vi "Create RPC Client Method.vi"(8 "error in (no error)":errorcluster, 10 "RPC Method Parameters":T1, 11 "Library":refnum<vi>) -> (0 "error out":errorcluster, 2 "Newly created ?":bool, 3 "Library":refnum<vi>)   [LabVIEW 2019, in "gRPC Template Creation Utility.lvlib"]
uses:
  gRPC Template Creation Utility.lvlib
  TypeDefs/RPC Method Parameters.ctl
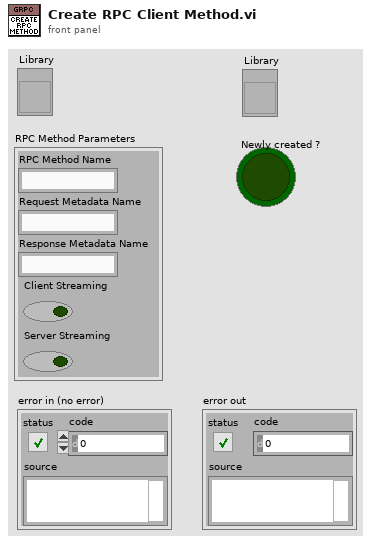
[diagram p1: front panel]
types:
  T1 = typedef "gRPC Template Creation Utility.lvlib/RPC Method Parameters.ctl" = cluster{"RPC Method Name":string, "Request Metadata Name":string, "Response Metadata Name":string, "Client Streaming":bool, "Server Streaming":bool}
  T2 = enum32{"invalid VI type", "Standard VI", "Control VI", "Global VI", "Polymorphic VI", "Configuration VI", "SubSystem", "Facade VI", "Method VI"}
  T3 = typedef "gRPC Template Creation Utility.lvlib/RPC Method Types.ctl" = enum16{"Unary", "Server Stream", "Client Stream", "Bidirectional Stream"}
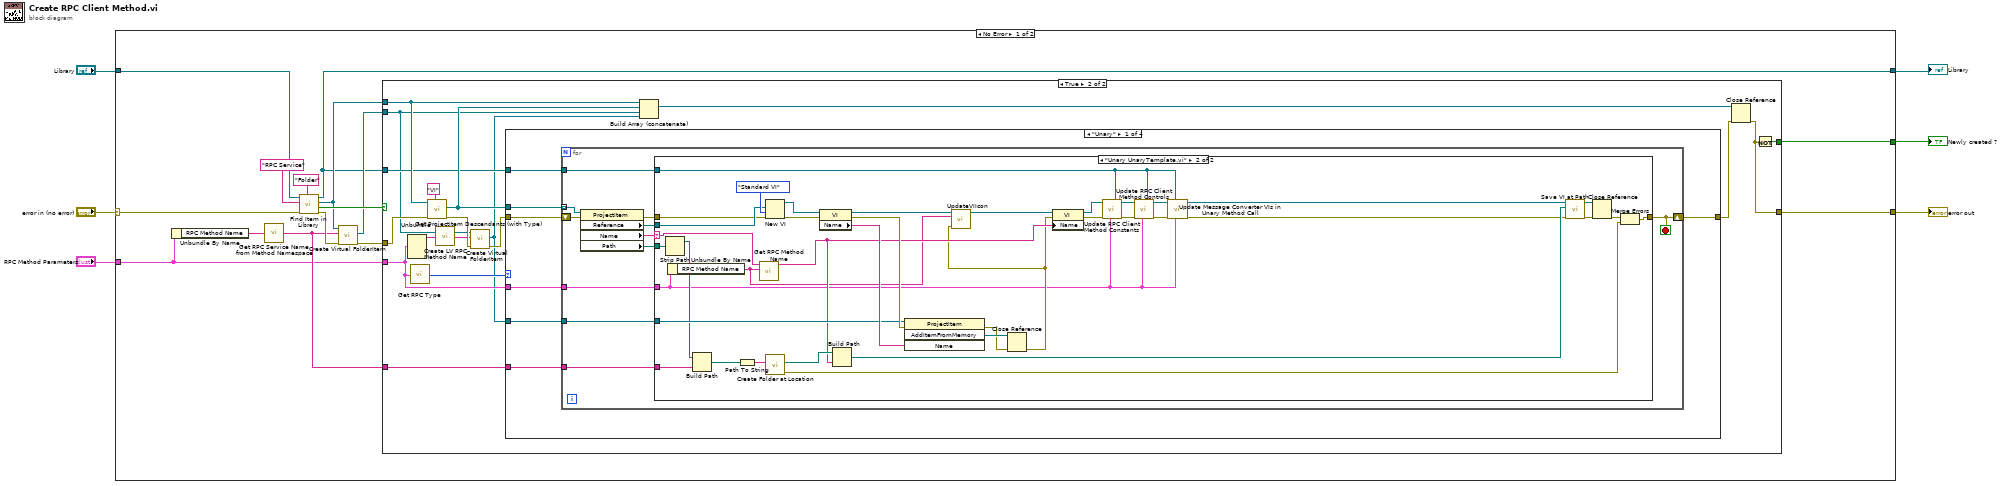
[diagram p0: block diagram]
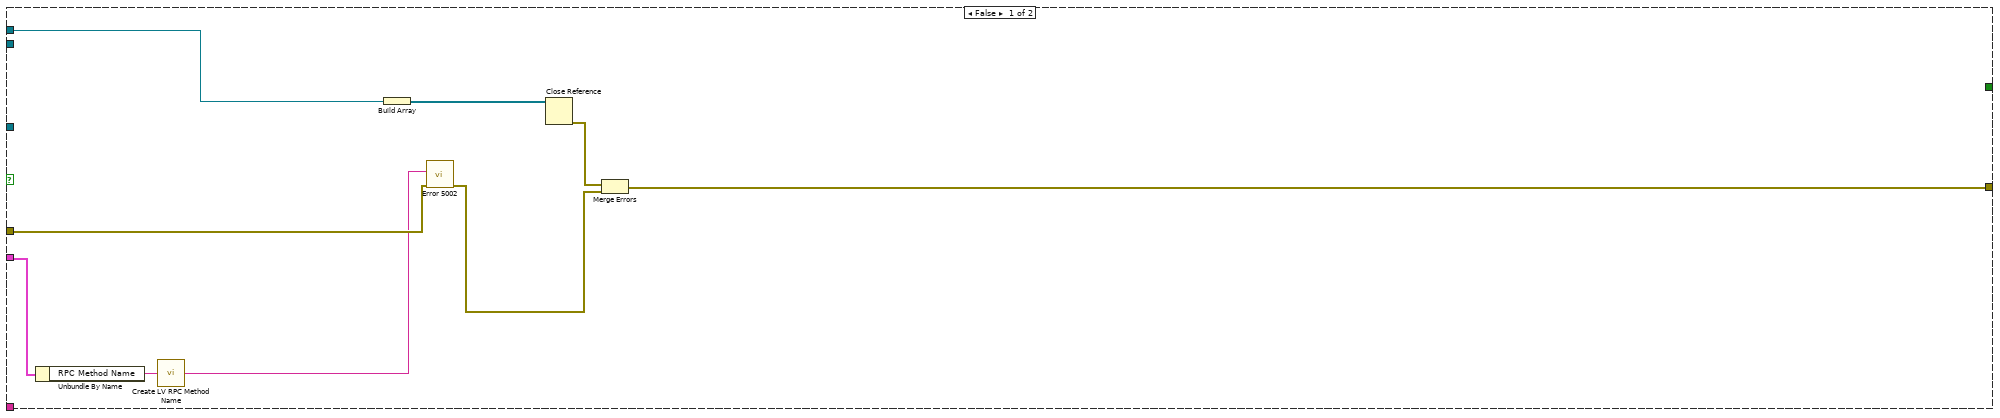
[diagram p2: hidden frame]
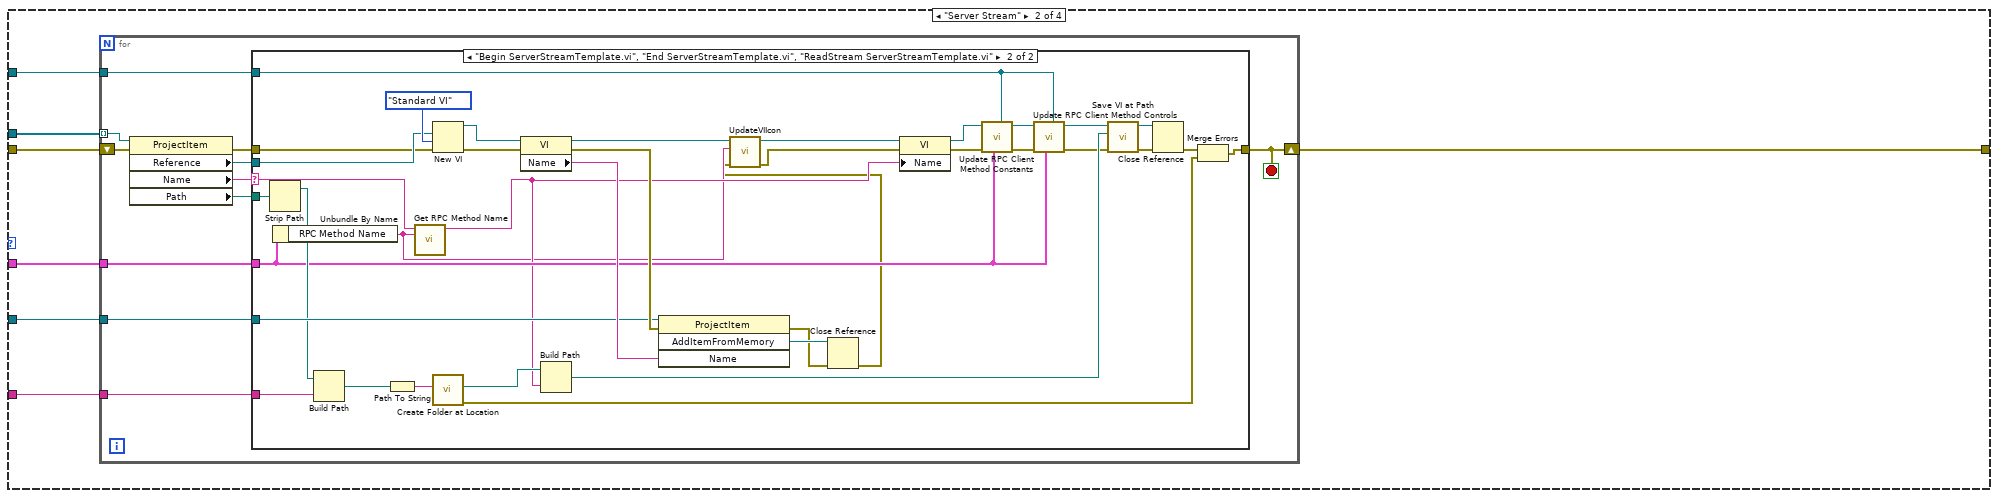
[diagram p4: hidden frame]
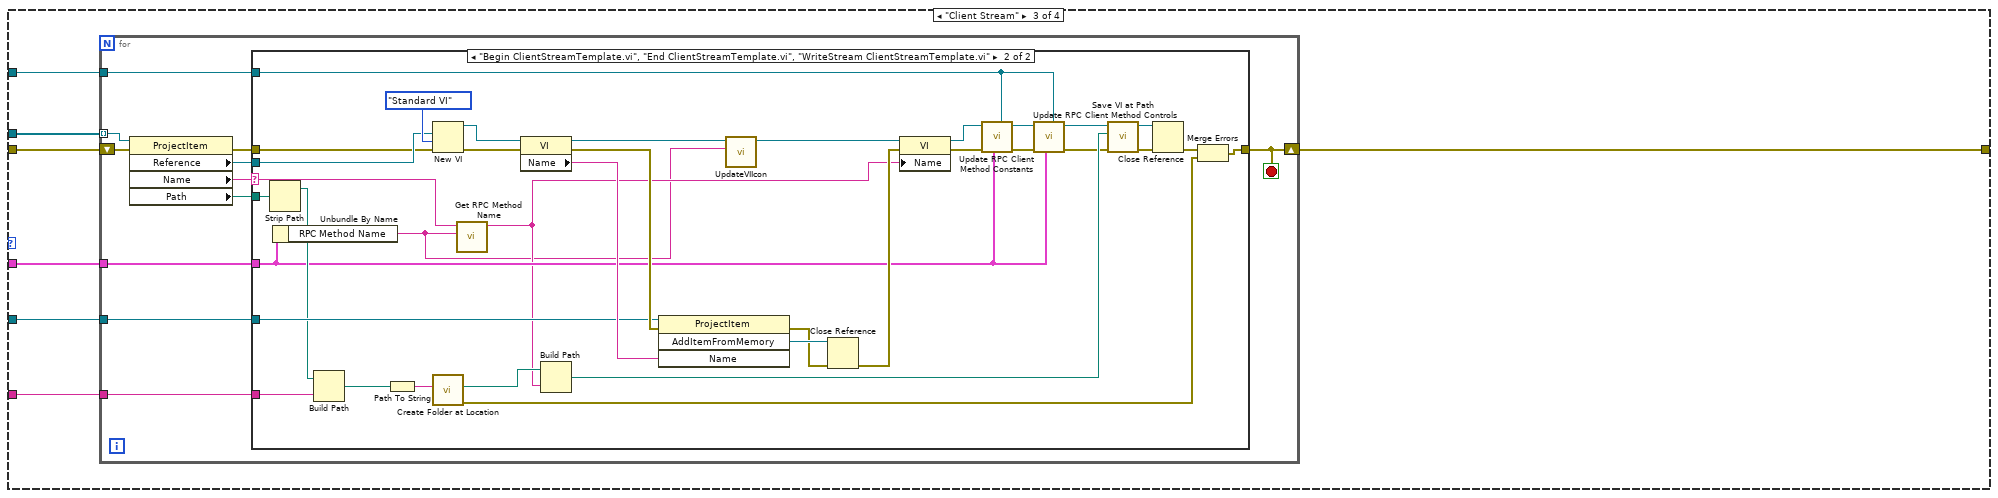
[diagram p6: hidden frame]
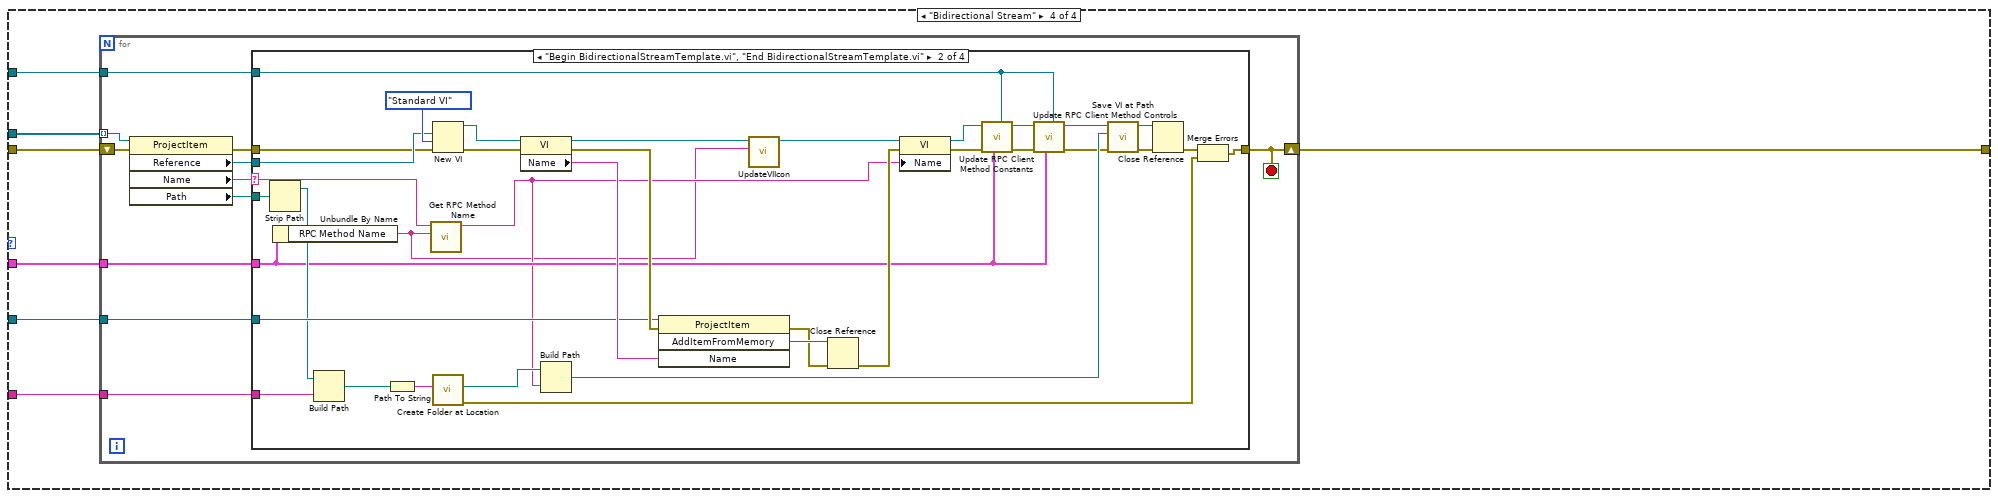
[diagram p8: hidden frame]
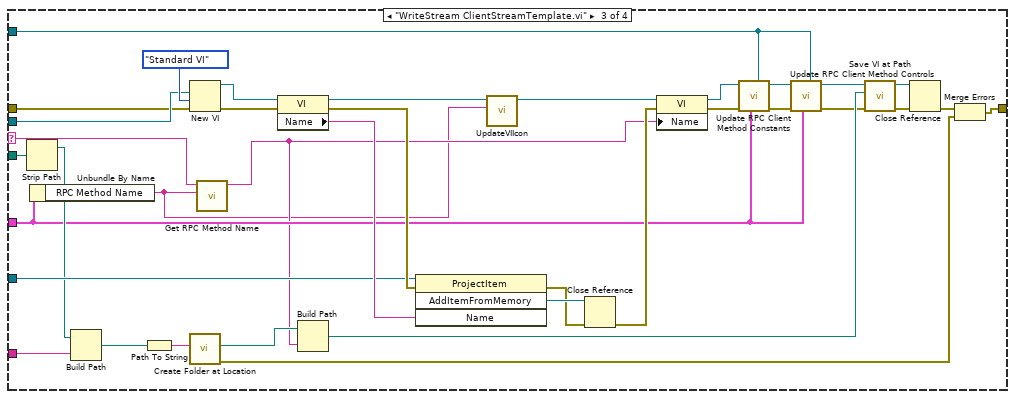
[diagram p10: hidden frame]
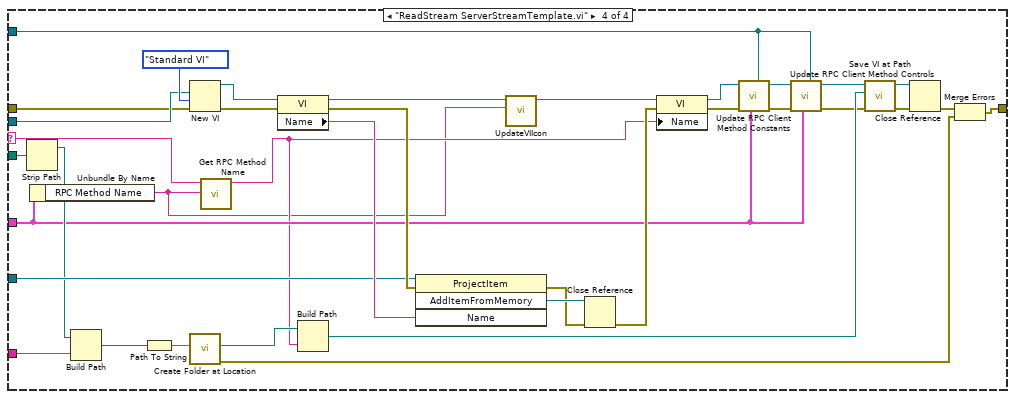
[diagram p11: hidden frame]
diagram:
  n1 = case shown="No Error" "error in (no error)" {
    selector: "error in (no error)" -> [w18 w345]
    tunnel: "Library" -> [w8 w344]
    tunnel: [w19 w345] -> w5
    tunnel: [w7 w344] -> w3
    tunnel: [w17 _] -> w2
    tunnel: "RPC Method Parameters" -> [w9 _]
    frame No Error {
      n2 = Unbundle By Name(w9) -> ("RPC Method Name"=w15:string)
      n3 = call "Get RPC Service Name from Method Namespace.vi"("RPC Method Name"=w15) -> ("RPC Service Name"=w10:string)
      n4 = call "Find Item in Library.vi"("Item Type"="Folder", "error in (no error)"=w18, "Item Name"="RPC Service", "Library item in"=w8) -> ("error out"=w14:errorcluster, "Found?"=w16:bool, "Project Item (Library Item)"=w12:refnum<vi>, "Library item out"=w7:refnum<vi>)  [unwired: 4 in]
      n5 = call "Create Virtual FolderItem.vi"("error in (no error)"=w14, "Folder Name"=w10, "ProjectItem in"=w12) -> ("error out"=w13:errorcluster, "FolderItem reference out"=w11:refnum<vi>)  [unwired: 5 in, 2 out]
      n6 = case shown="True" w16 {
        tunnel: w12 -> [w29 w41]
        tunnel: w13 -> [w30 w42]
        tunnel: [w25 w48] -> w19
        tunnel: [_ w47] -> w17
        tunnel: w11 -> [_ w35]
        tunnel: w10 -> [_ w40]
        tunnel: w9 -> [w24 w34]
        tunnel: w7 -> [_ w38]
        frame False {
          n7 = Unbundle By Name(w24) -> ("RPC Method Name"=w23:string)
          n8 = call "Create LV RPC Method Name.vi"("Proto Parser RPC Method Name in"=w23) -> ("LV RPC Method Name out"=w22:string)
          n9 = Build Array(w29) -> (w28:refnum<vi>[])
          n10 = call "Error 5002.vi"("error in (no error)"=w30, "Method Name"=w22) -> ("error out"=w27:errorcluster)  [unwired: 9 in]
          n11 = Close Reference(reference=w28) -> (error out=w26:errorcluster)  [unwired: 1 in]
          n12 = Merge Errors(w26, w27) -> (w25:errorcluster)
        }
        frame True {
          n13 = Unbundle(w34) -> ("RPC Method Name"=w32:string)  [unwired: 4 out]
          n14 = call "Get RPC Type.vi"("RPC Method Parameters"=w34) -> ("RPC Type"=w39:T3)
          n15 = call "Get ProjectItem Descendants (with Type).vi"("Type"="VI", "error in (no error)"=w42, "ProjectItem in"=w41) -> ("error out"=w37:errorcluster, "All Descendents"=w44:refnum<vi>[])  [unwired: 6 in, 1 out]
          n16 = call "Create LV RPC Method Name.vi"("Proto Parser RPC Method Name in"=w32) -> ("LV RPC Method Name out"=w31:string)
          n17 = call "Create Virtual FolderItem.vi"("error in (no error)"=w37, "Folder Name"=w31, "ProjectItem in"=w35) -> ("error out"=w36:errorcluster, "FolderItem reference out"=w33:refnum<vi>)  [unwired: 5 in, 2 out]
          n18 = case shown="\"Unary\"" w39 {
            tunnel: w44 -> [w55 w112 w168 w223]
            tunnel: w36 -> [w54 w111 w167 w222]
            tunnel: [w53 w110 w166 w221] -> w43
            tunnel: w33 -> [w52 w109 w165 w220]
            tunnel: w40 -> [w51 w108 w164 w219]
            tunnel: w34 -> [w50 w107 w163 w218]
            tunnel: w38 -> [w49 w106 w162 w217]
            frame "Unary" {
              n19 = for {
                tunnel: w55 -> [w66] mode=indexing
                tunnel: w52 -> [w61]
                shift-right: [w59] -> w53
                shift-left: w54 -> [w65]
                tunnel: w51 -> [w58]
                tunnel: w50 -> [w57]
                tunnel: w49 -> [w56]
                stop <- w59 stop-if-true
                n20 = property class="ProjectItem"(reference=w66, error in=w65) -> (error out=w60:errorcluster, "Reference"=w63:refnum<vi>, "Name"=w64:string, "Path"=w62:path)  [unwired: 1 out]
                n21 = case shown="\"Unary UnaryTemplate.vi\"" w64 {
                  selector: w64 -> [_ w79]
                  tunnel: w63 -> [_ w95]
                  tunnel: w62 -> [_ w91]
                  tunnel: w61 -> [_ w94]
                  tunnel: w60 -> [w67 w93]
                  tunnel: [w67 w85] -> w59
                  tunnel: w58 -> [_ w89]
                  tunnel: w57 -> [_ w69]
                  tunnel: w56 -> [_ w68]
                  frame "None", Default {
                  }
                  frame "Unary UnaryTemplate.vi" {
                    n22 = Strip Path(path=w91) -> (stripped path=w90:path)  [unwired: 1 out]
                    n23 = Unbundle By Name(w69) -> ("RPC Method Name"=w75:string)
                    n24 = Build Path(base path=w90, name or relative path=w89) -> (appended path=w88:path)
                    n25 = Path To String(path=w88) -> (string=w87:string)
                    n26 = call "Get RPC Method Name.vi"("RPC Method Name"=w75, "Template VI Name"=w79) -> ("RPC VI Name"=w78:string)  [unwired: 8 in, 1 out]
                    n27 = New VI(8:w93, 9:T2."Standard VI" ("vi type (standard vi)"), 10:w95) -> (0:w102:errorcluster, 3:w104:refnum<vi>)  [unwired: 1 in, 3 out]
                    n28 = call "Create Folder at Location.vi"("Path"=w87) -> ("Error Out"=w84:errorcluster, "Full path out"=w86:path)  [unwired: 8 in, 1 out]
                    n29 = property class="VI"(reference=w104, error in=w102) -> (reference out=w77:refnum<vi>, error out=w101:errorcluster, "Name"=w105:string)
                    n30 = Build Path(base path=w86, name or relative path=w78) -> (appended path=w100:path)
                    n31 = invoke class="ProjectItem" method="AddItemFromMemory"(reference=w94, error in=w101, "Name"=w105) -> (error out=w96:errorcluster, "AddItemFromMemory"=w97:refnum<vi>)  [unwired: 1 in, 2 out]
                    n32 = Close Reference(reference=w97, error in (no error)=w96) -> (error out=w74:errorcluster)
                    n33 = call "UpdateVIIcon.vi"("error in (no error)"=w74, "Method Name"=w75, "VI in"=w77) -> ("VI out"=w76:refnum<vi>)  [unwired: 7 in, 1 out]
                    n34 = property class="VI"(reference=w76, error in=w74, "Name"=w78) -> (reference out=w81:refnum<vi>, error out=w83:errorcluster)
                    n35 = call "Update RPC Client Method Constants.vi"("Library"=w68, "RPC Method Parameters"=w69, "error in (no error)"=w83, "VI in"=w81) -> ("error out"=w82:errorcluster, "VI out"=w80:refnum<vi>)  [unwired: 6 in]
                    n36 = call "Update RPC Client Method Controls.vi"("Library"=w68, "RPC Method Parameters"=w69, "error in (no error)"=w82, "VI in"=w80) -> ("error out"=w71:errorcluster, "VI out"=w73:refnum<vi>)  [unwired: 6 in]
                    n37 = call "Update Message Converter VIs in Unary Method Call.vi"("RPC Method Parameters"=w69, "Library"=w68, "error in (no error)"=w71, "VI in"=w73) -> ("error out"=w70:errorcluster, "VI out"=w72:refnum<vi>)  [unwired: 6 in]
                    n38 = call "Save VI at Path.vi"("error in (no error)"=w70, "Path"=w100, "VI in"=w72) -> ("error out"=w99:errorcluster, "VI out"=w98:refnum<vi>)  [unwired: 6 in, 1 out]
                    n39 = Close Reference(reference=w98, error in (no error)=w99) -> (error out=w92:errorcluster)
                    n40 = Merge Errors(w92, w84) -> (w85:errorcluster)
                  }
                }
              }
            }
            frame "Server Stream" {
              n41 = for {
                tunnel: w112 -> [w123] mode=indexing
                tunnel: w109 -> [w118]
                shift-right: [w116] -> w110
                shift-left: w111 -> [w122]
                tunnel: w108 -> [w115]
                tunnel: w107 -> [w114]
                tunnel: w106 -> [w113]
                stop <- w116 stop-if-true
                n42 = property class="ProjectItem"(reference=w123, error in=w122) -> (error out=w117:errorcluster, "Reference"=w120:refnum<vi>, "Name"=w121:string, "Path"=w119:path)  [unwired: 1 out]
                n43 = case shown="\"Begin ServerStreamTemplate.vi\", \"End ServerStreamTemplate.vi\", \"ReadStream ServerStreamTemplate.vi\"" w121 {
                  selector: w121 -> [_ w130]
                  tunnel: w120 -> [_ w151]
                  tunnel: w119 -> [_ w147]
                  tunnel: w118 -> [_ w150]
                  tunnel: w117 -> [w124 w149]
                  tunnel: [w124 w141] -> w116
                  tunnel: w115 -> [_ w145]
                  tunnel: w114 -> [_ w133]
                  tunnel: w113 -> [_ w132]
                  frame "None", Default {
                  }
                  frame "Begin ServerStreamTemplate.vi", "End ServerStreamTemplate.vi", "ReadStream ServerStreamTemplate.vi" {
                    n44 = Strip Path(path=w147) -> (stripped path=w146:path)  [unwired: 1 out]
                    n45 = Unbundle By Name(w133) -> ("RPC Method Name"=w127:string)
                    n46 = Build Path(base path=w146, name or relative path=w145) -> (appended path=w144:path)
                    n47 = Path To String(path=w144) -> (string=w143:string)
                    n48 = call "Get RPC Method Name.vi"("RPC Method Name"=w127, "Template VI Name"=w130) -> ("RPC VI Name"=w131:string)  [unwired: 8 in, 1 out]
                    n49 = New VI(8:w149, 9:T2."Standard VI" ("vi type (standard vi)"), 10:w151) -> (0:w158:errorcluster, 3:w160:refnum<vi>)  [unwired: 1 in, 3 out]
                    n50 = call "Create Folder at Location.vi"("Path"=w143) -> ("Error Out"=w140:errorcluster, "Full path out"=w142:path)  [unwired: 8 in, 1 out]
                    n51 = property class="VI"(reference=w160, error in=w158) -> (reference out=w129:refnum<vi>, error out=w157:errorcluster, "Name"=w161:string)
                    n52 = Build Path(base path=w142, name or relative path=w131) -> (appended path=w156:path)
                    n53 = invoke class="ProjectItem" method="AddItemFromMemory"(reference=w150, error in=w157, "Name"=w161) -> (error out=w152:errorcluster, "AddItemFromMemory"=w153:refnum<vi>)  [unwired: 1 in, 2 out]
                    n54 = Close Reference(reference=w153, error in (no error)=w152) -> (error out=w125:errorcluster)
                    n55 = call "UpdateVIIcon.vi"("error in (no error)"=w125, "Method Name"=w127, "VI in"=w129) -> ("error out"=w126:errorcluster, "VI out"=w128:refnum<vi>)  [unwired: 7 in]
                    n56 = property class="VI"(reference=w128, error in=w126, "Name"=w131) -> (reference out=w136:refnum<vi>, error out=w139:errorcluster)
                    n57 = call "Update RPC Client Method Constants.vi"("Library"=w132, "RPC Method Parameters"=w133, "error in (no error)"=w139, "VI in"=w136) -> ("error out"=w138:errorcluster, "VI out"=w135:refnum<vi>)  [unwired: 6 in]
                    n58 = call "Update RPC Client Method Controls.vi"("Library"=w132, "RPC Method Parameters"=w133, "error in (no error)"=w138, "VI in"=w135) -> ("error out"=w137:errorcluster, "VI out"=w134:refnum<vi>)  [unwired: 6 in]
                    n59 = call "Save VI at Path.vi"("error in (no error)"=w137, "Path"=w156, "VI in"=w134) -> ("error out"=w155:errorcluster, "VI out"=w154:refnum<vi>)  [unwired: 6 in, 1 out]
                    n60 = Close Reference(reference=w154, error in (no error)=w155) -> (error out=w148:errorcluster)
                    n61 = Merge Errors(w148, w140) -> (w141:errorcluster)
                  }
                }
              }
            }
            frame "Client Stream" {
              n62 = for {
                tunnel: w168 -> [w179] mode=indexing
                tunnel: w165 -> [w174]
                shift-right: [w172] -> w166
                shift-left: w167 -> [w178]
                tunnel: w164 -> [w171]
                tunnel: w163 -> [w170]
                tunnel: w162 -> [w169]
                stop <- w172 stop-if-true
                n63 = property class="ProjectItem"(reference=w179, error in=w178) -> (error out=w173:errorcluster, "Reference"=w176:refnum<vi>, "Name"=w177:string, "Path"=w175:path)  [unwired: 1 out]
                n64 = case shown="\"Begin ClientStreamTemplate.vi\", \"End ClientStreamTemplate.vi\", \"WriteStream ClientStreamTemplate.vi\"" w177 {
                  selector: w177 -> [_ w184]
                  tunnel: w176 -> [_ w205]
                  tunnel: w175 -> [_ w201]
                  tunnel: w174 -> [_ w204]
                  tunnel: w173 -> [w180 w203]
                  tunnel: [w180 w195] -> w172
                  tunnel: w171 -> [_ w199]
                  tunnel: w170 -> [_ w187]
                  tunnel: w169 -> [_ w186]
                  frame "None", Default {
                  }
                  frame "Begin ClientStreamTemplate.vi", "End ClientStreamTemplate.vi", "WriteStream ClientStreamTemplate.vi" {
                    n65 = Strip Path(path=w201) -> (stripped path=w200:path)  [unwired: 1 out]
                    n66 = Unbundle By Name(w187) -> ("RPC Method Name"=w181:string)
                    n67 = Build Path(base path=w200, name or relative path=w199) -> (appended path=w198:path)
                    n68 = Path To String(path=w198) -> (string=w197:string)
                    n69 = New VI(8:w203, 9:T2."Standard VI" ("vi type (standard vi)"), 10:w205) -> (0:w213:errorcluster, 3:w215:refnum<vi>)  [unwired: 1 in, 3 out]
                    n70 = call "Create Folder at Location.vi"("Path"=w197) -> ("Error Out"=w194:errorcluster, "Full path out"=w196:path)  [unwired: 8 in, 1 out]
                    n71 = call "Get RPC Method Name.vi"("RPC Method Name"=w181, "Template VI Name"=w184) -> ("RPC VI Name"=w185:string)  [unwired: 8 in, 1 out]
                    n72 = property class="VI"(reference=w215, error in=w213) -> (reference out=w183:refnum<vi>, error out=w212:errorcluster, "Name"=w216:string)
                    n73 = Build Path(base path=w196, name or relative path=w185) -> (appended path=w211:path)
                    n74 = invoke class="ProjectItem" method="AddItemFromMemory"(reference=w204, error in=w212, "Name"=w216) -> (error out=w207:errorcluster, "AddItemFromMemory"=w208:refnum<vi>)  [unwired: 1 in, 2 out]
                    n75 = call "UpdateVIIcon.vi"("Method Name"=w181, "VI in"=w183) -> ("VI out"=w182:refnum<vi>)  [unwired: 8 in, 1 out]
                    n76 = Close Reference(reference=w208, error in (no error)=w207) -> (error out=w206:errorcluster)
                    n77 = property class="VI"(reference=w182, error in=w206, "Name"=w185) -> (reference out=w190:refnum<vi>, error out=w193:errorcluster)
                    n78 = call "Update RPC Client Method Constants.vi"("Library"=w186, "RPC Method Parameters"=w187, "error in (no error)"=w193, "VI in"=w190) -> ("error out"=w192:errorcluster, "VI out"=w189:refnum<vi>)  [unwired: 6 in]
                    n79 = call "Update RPC Client Method Controls.vi"("Library"=w186, "RPC Method Parameters"=w187, "error in (no error)"=w192, "VI in"=w189) -> ("error out"=w191:errorcluster, "VI out"=w188:refnum<vi>)  [unwired: 6 in]
                    n80 = call "Save VI at Path.vi"("error in (no error)"=w191, "Path"=w211, "VI in"=w188) -> ("error out"=w210:errorcluster, "VI out"=w209:refnum<vi>)  [unwired: 6 in, 1 out]
                    n81 = Close Reference(reference=w209, error in (no error)=w210) -> (error out=w202:errorcluster)
                    n82 = Merge Errors(w202, w194) -> (w195:errorcluster)
                  }
                }
              }
            }
            frame "Bidirectional Stream" {
              n83 = for {
                tunnel: w223 -> [w234] mode=indexing
                tunnel: w220 -> [w229]
                shift-right: [w227] -> w221
                shift-left: w222 -> [w233]
                tunnel: w219 -> [w226]
                tunnel: w218 -> [w225]
                tunnel: w217 -> [w224]
                stop <- w227 stop-if-true
                n84 = property class="ProjectItem"(reference=w234, error in=w233) -> (error out=w228:errorcluster, "Reference"=w231:refnum<vi>, "Name"=w232:string, "Path"=w230:path)  [unwired: 1 out]
                n85 = case shown="\"Begin BidirectionalStreamTemplate.vi\", \"End BidirectionalStreamTemplate.vi\"" w232 {
                  selector: w232 -> [_ w239 w275 w311]
                  tunnel: w231 -> [_ w260 w296 w332]
                  tunnel: w230 -> [_ w256 w292 w328]
                  tunnel: w229 -> [_ w259 w295 w331]
                  tunnel: w228 -> [w235 w258 w294 w330]
                  tunnel: [w235 w250 w286 w322] -> w227
                  tunnel: w226 -> [_ w254 w290 w326]
                  tunnel: w225 -> [_ w242 w278 w314]
                  tunnel: w224 -> [_ w241 w277 w313]
                  frame "None", Default {
                  }
                  frame "Begin BidirectionalStreamTemplate.vi", "End BidirectionalStreamTemplate.vi" {
                    n86 = Strip Path(path=w256) -> (stripped path=w255:path)  [unwired: 1 out]
                    n87 = Unbundle By Name(w242) -> ("RPC Method Name"=w236:string)
                    n88 = Build Path(base path=w255, name or relative path=w254) -> (appended path=w253:path)
                    n89 = Path To String(path=w253) -> (string=w252:string)
                    n90 = call "Get RPC Method Name.vi"("RPC Method Name"=w236, "Template VI Name"=w239) -> ("RPC VI Name"=w240:string)  [unwired: 8 in, 1 out]
                    n91 = New VI(8:w258, 9:T2."Standard VI" ("vi type (standard vi)"), 10:w260) -> (0:w268:errorcluster, 3:w270:refnum<vi>)  [unwired: 1 in, 3 out]
                    n92 = call "Create Folder at Location.vi"("Path"=w252) -> ("Error Out"=w249:errorcluster, "Full path out"=w251:path)  [unwired: 8 in, 1 out]
                    n93 = property class="VI"(reference=w270, error in=w268) -> (reference out=w238:refnum<vi>, error out=w267:errorcluster, "Name"=w271:string)
                    n94 = Build Path(base path=w251, name or relative path=w240) -> (appended path=w266:path)
                    n95 = invoke class="ProjectItem" method="AddItemFromMemory"(reference=w259, error in=w267, "Name"=w271) -> (error out=w262:errorcluster, "AddItemFromMemory"=w263:refnum<vi>)  [unwired: 1 in, 2 out]
                    n96 = call "UpdateVIIcon.vi"("Method Name"=w236, "VI in"=w238) -> ("VI out"=w237:refnum<vi>)  [unwired: 8 in, 1 out]
                    n97 = Close Reference(reference=w263, error in (no error)=w262) -> (error out=w261:errorcluster)
                    n98 = property class="VI"(reference=w237, error in=w261, "Name"=w240) -> (reference out=w245:refnum<vi>, error out=w248:errorcluster)
                    n99 = call "Update RPC Client Method Constants.vi"("Library"=w241, "RPC Method Parameters"=w242, "error in (no error)"=w248, "VI in"=w245) -> ("error out"=w247:errorcluster, "VI out"=w244:refnum<vi>)  [unwired: 6 in]
                    n100 = call "Update RPC Client Method Controls.vi"("Library"=w241, "RPC Method Parameters"=w242, "error in (no error)"=w247, "VI in"=w244) -> ("error out"=w246:errorcluster, "VI out"=w243:refnum<vi>)  [unwired: 6 in]
                    n101 = call "Save VI at Path.vi"("error in (no error)"=w246, "Path"=w266, "VI in"=w243) -> ("error out"=w265:errorcluster, "VI out"=w264:refnum<vi>)  [unwired: 6 in, 1 out]
                    n102 = Close Reference(reference=w264, error in (no error)=w265) -> (error out=w257:errorcluster)
                    n103 = Merge Errors(w257, w249) -> (w250:errorcluster)
                  }
                  frame "WriteStream ClientStreamTemplate.vi" {
                    n104 = Strip Path(path=w292) -> (stripped path=w291:path)  [unwired: 1 out]
                    n105 = Unbundle By Name(w278) -> ("RPC Method Name"=w272:string)
                    n106 = Build Path(base path=w291, name or relative path=w290) -> (appended path=w289:path)
                    n107 = Path To String(path=w289) -> (string=w288:string)
                    n108 = New VI(8:w294, 9:T2."Standard VI" ("vi type (standard vi)"), 10:w296) -> (0:w304:errorcluster, 3:w306:refnum<vi>)  [unwired: 1 in, 3 out]
                    n109 = call "Create Folder at Location.vi"("Path"=w288) -> ("Error Out"=w285:errorcluster, "Full path out"=w287:path)  [unwired: 8 in, 1 out]
                    n110 = call "Get RPC Method Name.vi"("RPC Method Name"=w272, "Template VI Name"=w275) -> ("RPC VI Name"=w276:string)  [unwired: 8 in, 1 out]
                    n111 = property class="VI"(reference=w306, error in=w304) -> (reference out=w274:refnum<vi>, error out=w303:errorcluster, "Name"=w307:string)
                    n112 = Build Path(base path=w287, name or relative path=w276) -> (appended path=w302:path)
                    n113 = invoke class="ProjectItem" method="AddItemFromMemory"(reference=w295, error in=w303, "Name"=w307) -> (error out=w298:errorcluster, "AddItemFromMemory"=w299:refnum<vi>)  [unwired: 1 in, 2 out]
                    n114 = call "UpdateVIIcon.vi"("Method Name"=w272, "VI in"=w274) -> ("VI out"=w273:refnum<vi>)  [unwired: 8 in, 1 out]
                    n115 = Close Reference(reference=w299, error in (no error)=w298) -> (error out=w297:errorcluster)
                    n116 = property class="VI"(reference=w273, error in=w297, "Name"=w276) -> (reference out=w281:refnum<vi>, error out=w284:errorcluster)
                    n117 = call "Update RPC Client Method Constants.vi"("Library"=w277, "RPC Method Parameters"=w278, "error in (no error)"=w284, "VI in"=w281) -> ("error out"=w283:errorcluster, "VI out"=w280:refnum<vi>)  [unwired: 6 in]
                    n118 = call "Update RPC Client Method Controls.vi"("Library"=w277, "RPC Method Parameters"=w278, "error in (no error)"=w283, "VI in"=w280) -> ("error out"=w282:errorcluster, "VI out"=w279:refnum<vi>)  [unwired: 6 in]
                    n119 = call "Save VI at Path.vi"("error in (no error)"=w282, "Path"=w302, "VI in"=w279) -> ("error out"=w301:errorcluster, "VI out"=w300:refnum<vi>)  [unwired: 6 in, 1 out]
                    n120 = Close Reference(reference=w300, error in (no error)=w301) -> (error out=w293:errorcluster)
                    n121 = Merge Errors(w293, w285) -> (w286:errorcluster)
                  }
                  frame "ReadStream ServerStreamTemplate.vi" {
                    n122 = Strip Path(path=w328) -> (stripped path=w327:path)  [unwired: 1 out]
                    n123 = Unbundle By Name(w314) -> ("RPC Method Name"=w308:string)
                    n124 = Build Path(base path=w327, name or relative path=w326) -> (appended path=w325:path)
                    n125 = Path To String(path=w325) -> (string=w324:string)
                    n126 = New VI(8:w330, 9:T2."Standard VI" ("vi type (standard vi)"), 10:w332) -> (0:w340:errorcluster, 3:w342:refnum<vi>)  [unwired: 1 in, 3 out]
                    n127 = call "Create Folder at Location.vi"("Path"=w324) -> ("Error Out"=w321:errorcluster, "Full path out"=w323:path)  [unwired: 8 in, 1 out]
                    n128 = call "Get RPC Method Name.vi"("RPC Method Name"=w308, "Template VI Name"=w311) -> ("RPC VI Name"=w312:string)  [unwired: 8 in, 1 out]
                    n129 = property class="VI"(reference=w342, error in=w340) -> (reference out=w310:refnum<vi>, error out=w339:errorcluster, "Name"=w343:string)
                    n130 = Build Path(base path=w323, name or relative path=w312) -> (appended path=w338:path)
                    n131 = invoke class="ProjectItem" method="AddItemFromMemory"(reference=w331, error in=w339, "Name"=w343) -> (error out=w334:errorcluster, "AddItemFromMemory"=w335:refnum<vi>)  [unwired: 1 in, 2 out]
                    n132 = call "UpdateVIIcon.vi"("Method Name"=w308, "VI in"=w310) -> ("VI out"=w309:refnum<vi>)  [unwired: 8 in, 1 out]
                    n133 = Close Reference(reference=w335, error in (no error)=w334) -> (error out=w333:errorcluster)
                    n134 = property class="VI"(reference=w309, error in=w333, "Name"=w312) -> (reference out=w317:refnum<vi>, error out=w320:errorcluster)
                    n135 = call "Update RPC Client Method Constants.vi"("Library"=w313, "RPC Method Parameters"=w314, "error in (no error)"=w320, "VI in"=w317) -> ("error out"=w319:errorcluster, "VI out"=w316:refnum<vi>)  [unwired: 6 in]
                    n136 = call "Update RPC Client Method Controls.vi"("Library"=w313, "RPC Method Parameters"=w314, "error in (no error)"=w319, "VI in"=w316) -> ("error out"=w318:errorcluster, "VI out"=w315:refnum<vi>)  [unwired: 6 in]
                    n137 = call "Save VI at Path.vi"("error in (no error)"=w318, "Path"=w338, "VI in"=w315) -> ("error out"=w337:errorcluster, "VI out"=w336:refnum<vi>)  [unwired: 6 in, 1 out]
                    n138 = Close Reference(reference=w336, error in (no error)=w337) -> (error out=w329:errorcluster)
                    n139 = Merge Errors(w329, w321) -> (w322:errorcluster)
                  }
                }
              }
            }
          }
          n140 = Build Array (concatenate)(w41, w44, w35, w33) -> (w46:refnum<vi>[])
          n141 = Close Reference(reference=w46, error in (no error)=w43) -> (error out=w48:errorcluster)
          n142 = Not(x=w48) -> (.not. x?=w47:bool)
        }
      }
    }
    frame Error {
    }
  }
  "error out" <- w5
  "Library" <- w3
  "Newly created ?" <- w2
